vi "弹窗-浮动数字键盘.vi"(11 "引用-文本框":refnum<vi>) -> ()   [LabVIEW 2013]
uses:
  <vilib>/Utility/miscctls.llb/LVSelectionTypeDef.ctl
panel:
  in  "停止？":bool=TRUE
  in  "延迟次数":i32
  in  "输入框":string
  in  "1":bool
  in  "2":bool
  in  "3":bool
  in  "4":bool
  in  "5":bool
  in  "6":bool
  in  "7":bool
  in  "8":bool
  in  "9":bool
  in  "DEL":bool
  in  "0":bool
  in  "确定":bool
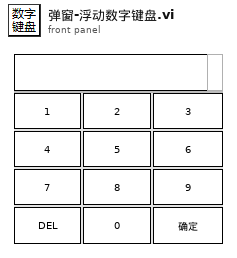
[diagram p1: front panel]
types:
  T1 = enum32{"Invalid", "Standard", "Closed", "Hidden", "Minimized", "Maximized"}
  T2 = typedef "LVSelectionTypeDef.ctl" = cluster{"Selection Start":u32, "Selection End":u32}
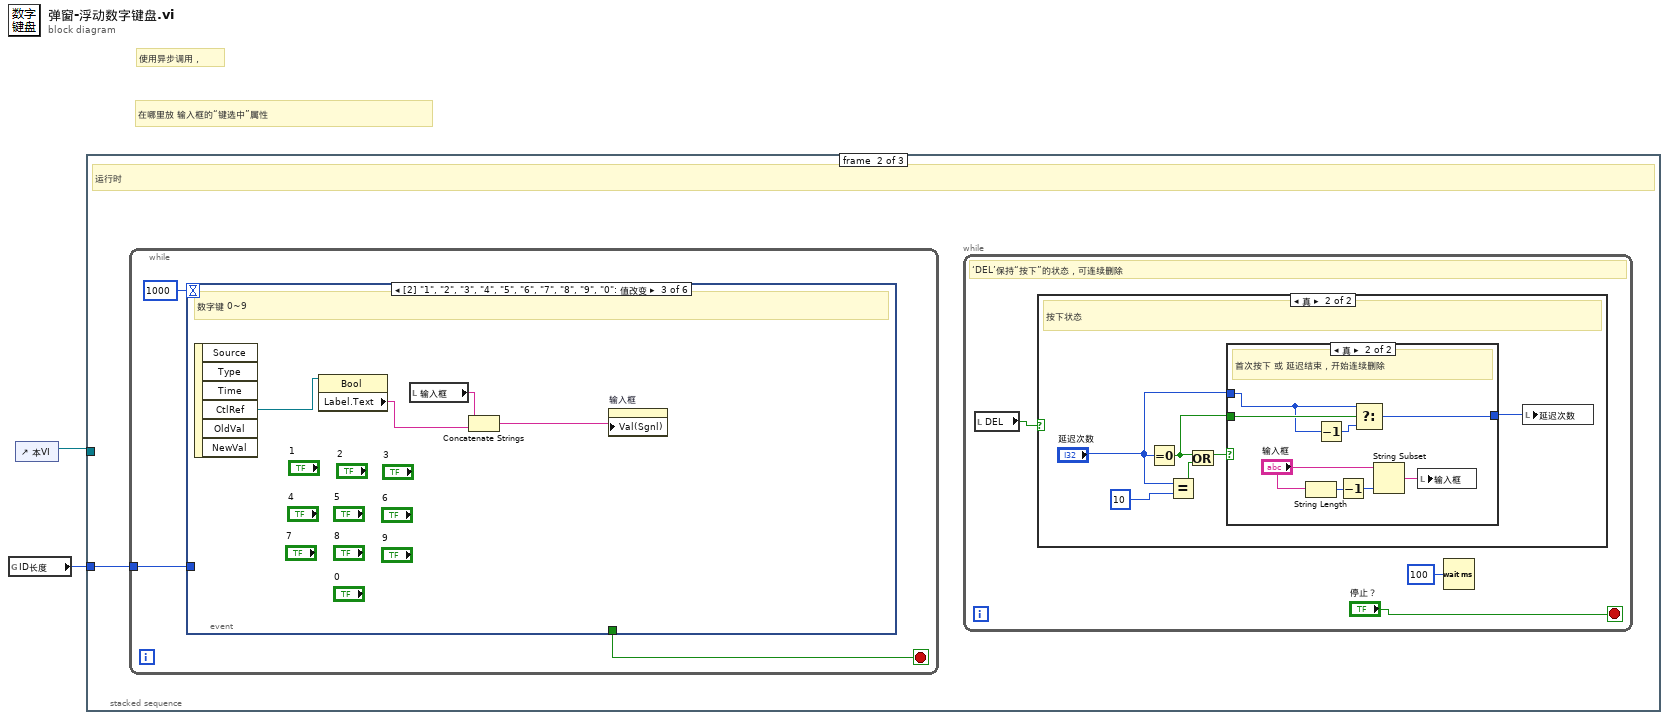
[diagram p0: block diagram]
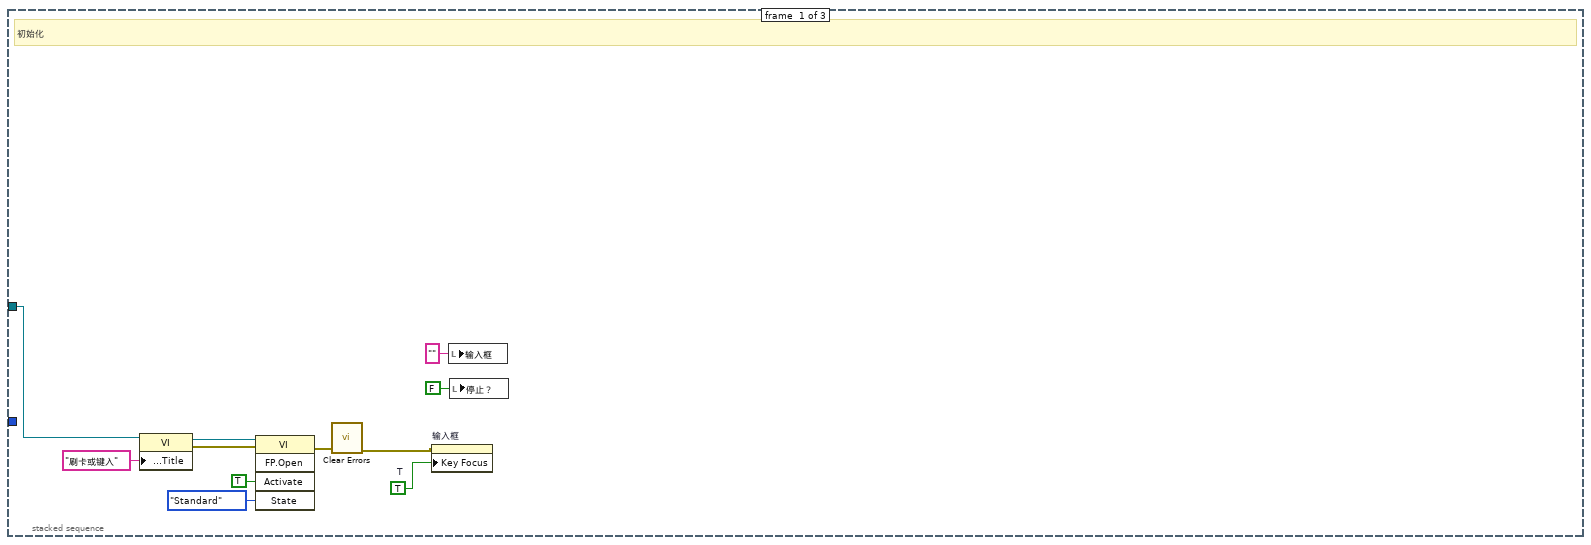
[diagram p2: hidden frame]
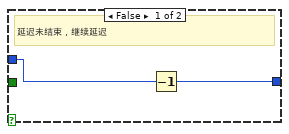
[diagram p4: hidden frame]
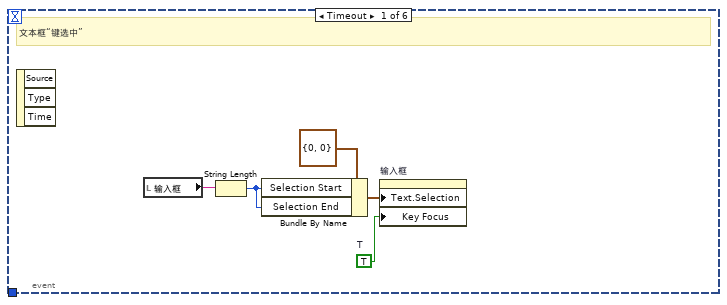
[diagram p5: hidden frame]
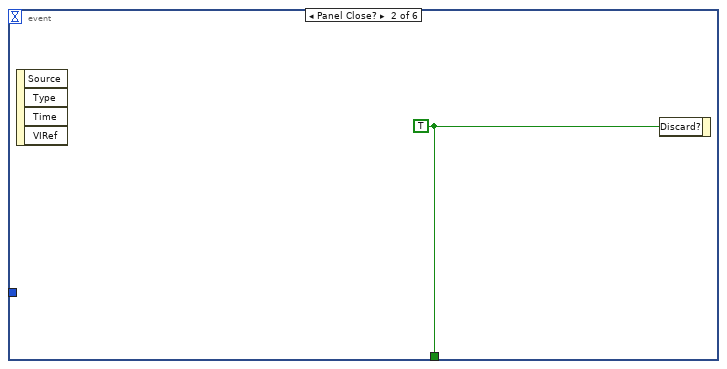
[diagram p6: hidden frame]
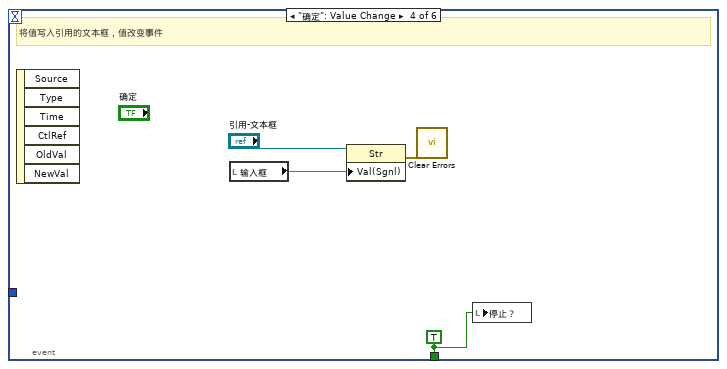
[diagram p7: hidden frame]
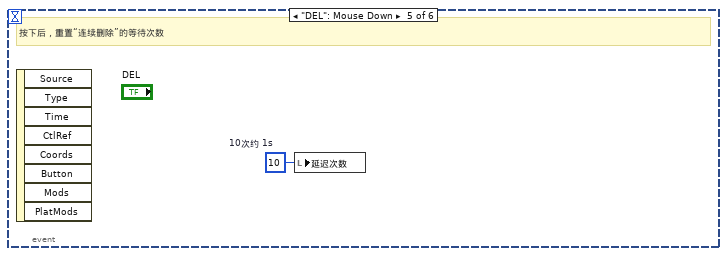
[diagram p8: hidden frame]
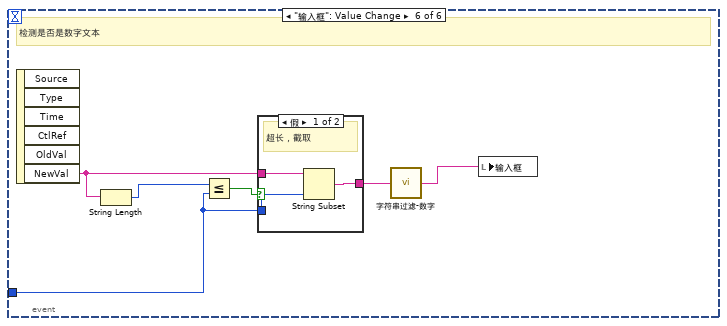
[diagram p9: hidden frame]
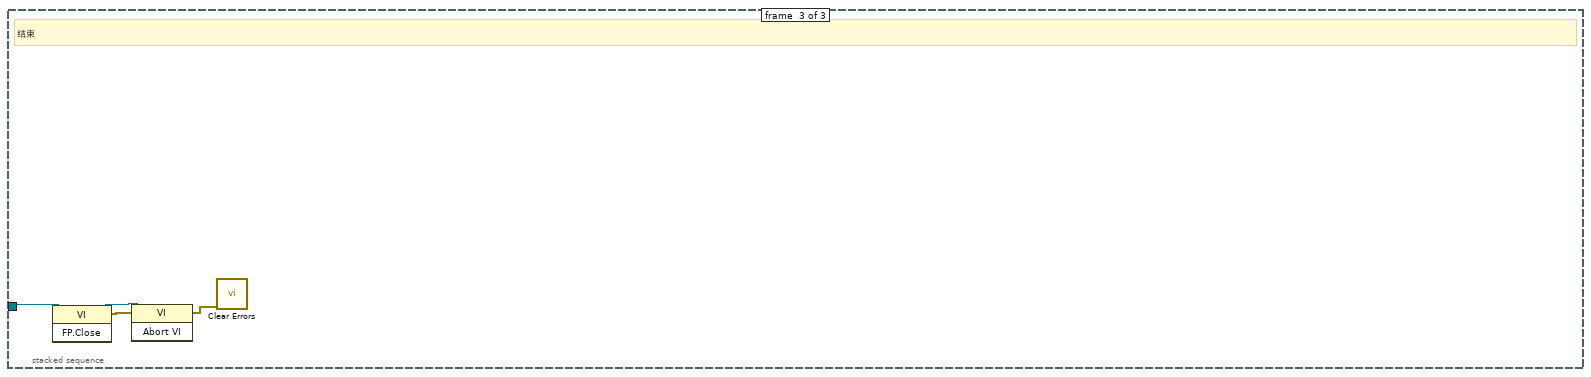
[diagram p11: hidden frame]
diagram:
  # "使用异步调用，"
  # "在哪里放 输入框的“键选中”属性"
  n1 = global read "全局变量-手足.vi" "ID长度"() -> (w1:i32)
  n2 = control-ref of="本VI"() -> (w2:refnum<vi>)
  n3 = stacked-sequence {
    tunnel: w2 -> [w13 _ w65]
    tunnel: w1 -> [_ w14 _]
    frame #0 {
      w5 = TRUE  # T
      # "初始化"
      n4 = property class="VI"(reference=w13, "Front Panel.Title"="刷卡或键入" ("前面板窗口:标题")) -> (reference out=w11:refnum<vi>, error out=w10:errorcluster)  [unwired: 1 in]
      n5 = invoke class="VI" method="FP.Open"(reference=w11, error in=w10, "Activate"=TRUE ("激活？"), "State"=T1."Standard" ("状态")) -> (error out=w7:errorcluster)  [unwired: 1 in, 4 out]
      n6 = call <vilib>:"Clear Errors.vi"("error in (no error)"=w7) -> ("error out"=w6:errorcluster)  [unwired: 6 in]
      n7 = property on="输入框" class="Str"(error in=w6, "Key Focus"=w5) -> ()  [unwired: 1 in, 2 out]
      n8 = local write "输入框"("" ("输入框")) -> ()
      n9 = local write "停止？"(FALSE ("停止？")) -> ()
    }
    frame #1 {
      # "运行时"
      n10 = while {
        tunnel: w14 -> [w34]
        stop <- w36 stop-if-true
        n11 = event shown="[2] \"1\", \"2\", \"3\", \"4\", \"5\", \"6\", \"7\", \"8\", \"9\", \"0\": 值改变" {
          selector: _ -> [_ _ _ _ _ _]
          dyn-events: _ -> [_ _ _ _ _ _]
          timeout: 1000 -> [_ _ _ _ _ _]
          tunnel: [_ w42 _ w47 _ _] -> w36
          tunnel: w34 -> [_ _ _ _ _ w54]
          event Timeout {
            w41 = TRUE  # T
            # "文本框“键选中”"
            n12 = event-data() -> ()  [unwired: 1 in, 3 out]
            n13 = local read "输入框"() -> (w38:string)
            n14 = String Length(string=w38) -> (length=w37:i32)
            n15 = Bundle By Name(cluster=T2 {"Selection Start"=0, "Selection End"=0} ("文本.选择"), "Selection Start"=w37, "Selection End"=w37) -> (w39:T2)
            n16 = property on="输入框" class="Str"("Text.Selection"=w39, "Key Focus"=w41) -> ()  [unwired: 2 in, 2 out]
          }
          event Panel Close? {
            w42 = TRUE ("放弃？")
            n17 = event-data() -> ()  [unwired: 1 in, 4 out]
            n18 = event-data("Discard?"=w42) -> ()  [unwired: 1 in, 1 out]
          }
          event "1", "2", "3", "4", "5", "6", "7", "8", "9", "0": Value Change {
            # "数字键 0~9"
            n19 = event-data() -> ("CtlRef"=w46:refnum<vi>)  [unwired: 1 in, 5 out]
            n20 = property class="Bool"(reference=w46) -> ("Label.Text"=w44:string)  [unwired: 1 in, 2 out]
            n21 = local read "输入框"() -> (w45:string)
            n22 = Concatenate Strings(w45, w44) -> (w43:string)
            n23 = property on="输入框" class="Str"("Val(Sgnl)"=w43) -> ()  [unwired: 2 in, 2 out]
          }
          event "确定": Value Change {
            w47 = TRUE ("放弃？")
            # "将值写入引用的文本框，值改变事件"
            n24 = event-data() -> ()  [unwired: 1 in, 6 out]
            n25 = local read "输入框"() -> (w49:string)
            n26 = property class="Str"(reference="引用-文本框", "Val(Sgnl)"=w49) -> (error out=w48:errorcluster)  [unwired: 1 in, 1 out]
            n27 = call <vilib>:"Clear Errors.vi"("error in (no error)"=w48) -> ()  [unwired: 6 in, 1 out]
            n28 = local write "停止？"(w47) -> ()
          }
          event "DEL": Mouse Down {
            w51 = 10  # 10次约 1s
            # "按下后，重置“连续删除”的等待次数"
            n29 = event-data() -> ()  [unwired: 1 in, 8 out]
            n30 = local write "延迟次数"(w51) -> ()
          }
          event "输入框": Value Change {
            # "检测是否是数字文本"
            n31 = event-data() -> ("NewVal"=w53:string)  [unwired: 1 in, 5 out]
            n32 = String Length(string=w53) -> (length=w56:i32)
            n33 = Less Or Equal?(x=w56, y=w54) -> (x <= y?=w55:bool)
            n34 = case shown="假" w55 {
              tunnel: w54 -> [w59 _]
              tunnel: w53 -> [w60 w61]
              tunnel: [w58 w61] -> w52
              frame False {
                # "超长，截取"
                n35 = String Subset(string=w60, length (rest)=w59) -> (substring=w58:string)  [unwired: 1 in]
              }
              frame True {
              }
            }
            n36 = call "字符串过滤-数字.vi"("字符串 i"=w52) -> ("字符串 o"=w57:string)  [unwired: 3 in, 1 out]
            n37 = local write "输入框"(w57) -> ()
          }
        }
      }
      n38 = while {
        stop <- "停止？" stop-if-true
        # "‘DEL’保持“按下”的状态，可连续删除"
        n39 = local read "DEL"() -> (w15:bool)
        n40 = case shown="真" w15 {
          frame False {
            # "没有按下"
          }
          frame True {
            # "按下状态"
            n41 = Equal To 0?(x="延迟次数") -> (x = 0?=w19:bool)
            n42 = Equal?(x="延迟次数", y=10) -> (x = y?=w23:bool)
            n43 = Or(x=w19, y=w23) -> (x .or. y?=w22:bool)
            n44 = case shown="真" w22 {
              tunnel: "延迟次数" -> [w25 w28]
              tunnel: w19 -> [_ w29]
              tunnel: [w24 w26] -> w18
              frame False {
                # "延迟未结束，继续延迟"
                n45 = Decrement(x=w25) -> (x-1=w24:i32)
              }
              frame True {
                # "首次按下 或 延迟结束，开始连续删除"
                n46 = String Length(string="输入框") -> (length=w32:i32)
                n47 = Decrement(x=w28) -> (x-1=w27:i32)
                n48 = Decrement(x=w32) -> (x-1=w31:i32)
                n49 = Select(t=w28, s=w29, f=w27) -> (s? t:f=w26:i32)
                n50 = String Subset(string="输入框", length (rest)=w31) -> (substring=w30:string)  [unwired: 1 in]
                n51 = local write "输入框"(w30) -> ()
              }
            }
            n52 = local write "延迟次数"(w18) -> ()
          }
        }
        n53 = Wait (ms)(milliseconds to wait=u32 100 ("等待时间（毫秒）")) -> ()  [unwired: 1 out]
      }
    }
    frame #2 {
      # "结束"
      n54 = invoke class="VI" method="FP.Close"(reference=w65) -> (reference out=w63:refnum<vi>, error out=w64:errorcluster)  [unwired: 2 in, 1 out]
      n55 = invoke class="VI" method="Abort VI"(reference=w63, error in=w64) -> (error out=w62:errorcluster)  [unwired: 1 in, 2 out]
      n56 = call <vilib>:"Clear Errors.vi"("error in (no error)"=w62) -> ()  [unwired: 6 in, 1 out]
    }
  }
